vi "Run Test Application.vi"(8 "error in (no error)":errorcluster, 10 "Tests":refnum<class "Test Class.lvclass">[](array[class]), 11 "Application Template in":refnum<class "Example Application.lvclass">) -> (0 "error out":errorcluster, 3 "Application Template out":refnum<class "Example Application.lvclass">)   [LabVIEW 2015, in "Example Application.lvlib" / "Example Application.lvclass"]
uses:
  Example Application.lvclass
  CBTF Modules/Tests/Tests/Examples/Example Test/Example Test.lvclass
  CBTF Modules/Classes/Application/Class/Application.lvclass
  CBTF Modules/Tests/Test Class/Test Class.lvclass
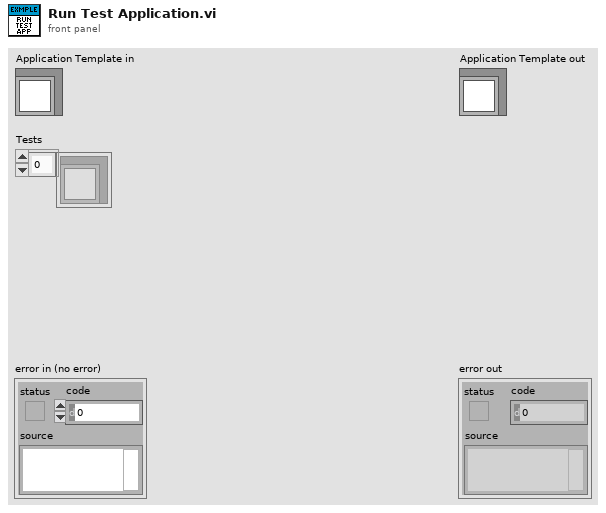
[diagram p1: front panel]
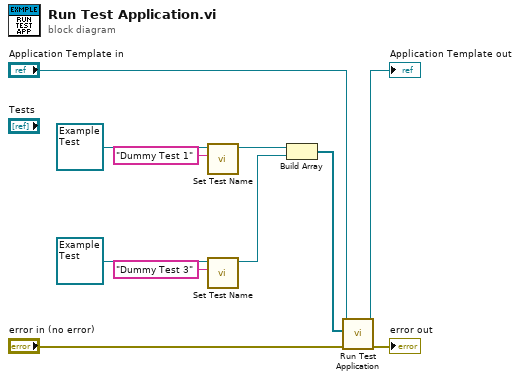
[diagram p0: block diagram]
diagram:
  n1 = call "Set Test Name.vi"("Test Name"="Dummy Test 1", "Test Class in"=refnum<class "Example Test.lvclass"> refnum ("Example Test.lvclass")) -> ("Test Class out"=w5:refnum<class "Example Test.lvclass">)  [unwired: 8 in, 1 out]
  n2 = call "Set Test Name.vi"("Test Name"="Dummy Test 3", "Test Class in"=refnum<class "Example Test.lvclass"> refnum ("Example Test.lvclass")) -> ("Test Class out"=w1:refnum<class "Example Test.lvclass">)  [unwired: 8 in, 1 out]
  n3 = Build Array(w5, w1) -> (w7:refnum<class "Example Test.lvclass">[])
  n4 = call-parent "Run Test Application.vi"("error in (no error)"="error in (no error)", "Tests"=w7, "Application in"="Application Template in") -> ("error out"=→"error out":errorcluster, "Application out"=→"Application Template out":refnum<class "Example Application.lvclass">)  [unwired: 7 in]
